vi "Chart.vi"() -> (7 "Waveform Chart":dbl(graph))   [LabVIEW 2020]
doc: "This system is a subVI which is used to plot the data as per the value change in the slider in the main system"
panel:
  out "Error out":errorcluster
  in  "Error in":errorcluster
  # "Chart to Display data"
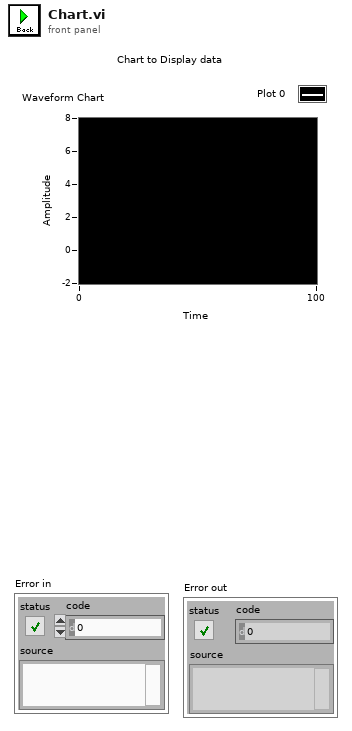
[diagram p1: front panel]
types:
  T1 = enum16{"Get Ref", "Destroy", "Create", "Generate"}
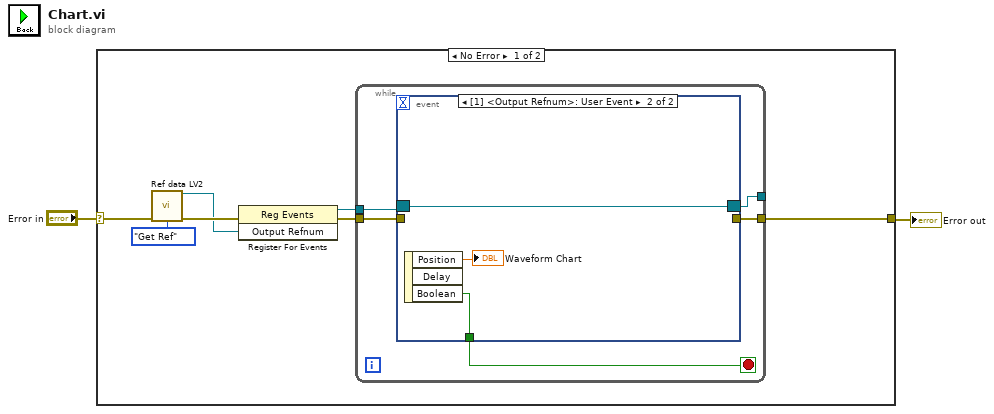
[diagram p0: block diagram]
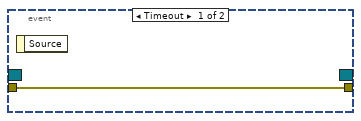
[diagram p2: hidden frame]
diagram:
  n1 = case shown="No Error" "Error in" {
    selector: "Error in" -> [w7 w19]
    tunnel: [w3 w19] -> w1
    frame No Error {
      n2 = call "Ref data LV2.vi"("error in"=w7, "Enum"=T1."Get Ref") -> ("Output Refnum"=w4:refnum<user-event>, "error out"=w9:errorcluster)  [unwired: 12 in]
      n3 = register-events(error in=w9, w4) -> (reference out=w5:refnum<event-registration>, error out=w6:errorcluster)  [unwired: 1 in]
      n4 = while {
        tunnel: w6 -> [w14]
        tunnel: [w13] -> w3
        tunnel: w5 -> [w12]
        tunnel: [w11] -> _
        stop <- w10 stop-if-true
        n5 = event shown="[1] <Output Refnum>: User Event" {
          selector: w12 -> [_ w17]
          dyn-events: [_ w17] -> w11
          timeout: _ -> [_ _]
          tunnel: w14 -> [w15 _]
          tunnel: [w15 _] -> w13
          tunnel: [_ w16] -> w10
          event Timeout {
            n6 = event-data() -> ()  [unwired: 1 in, 1 out]
          }
          event User Event {
            n7 = event-data() -> ("Position"=→"Waveform Chart":dbl, "Boolean"=w16:bool)  [unwired: 1 in, 1 out]
          }
        }
      }
    }
    frame Error {
    }
  }
  "Error out" <- w1
